vi "svfa_Mag to Mag2.vi"(0 "input signal":dbl[](array[numeric]) format="%.2f", 1 "power/magnitude desired":enum16{"no change", "power", "magnitude"}(ring), 5 "linear/dB":enum16{"linear", "dB"}(ring), 7 "power/magnitude":enum16{"power", "magnitude"}(ring), 9 "view":enum16{"rms", "peak", "peak-peak"}(ring), 11 "dB reference":dbl format="%.2f") -> (4 "converted signal":dbl[](array[numeric]) format="%.2f", 6 "dup linear/dB":enum16{"linear", "dB"}(ring), 8 "power/magnitude (out)":enum16{"power", "magnitude"}(ring), 10 "dup view":enum16{"rms", "peak", "peak-peak"}(ring), 15 "dB reference (out)":dbl format="%.2f")   [LabVIEW 2017]
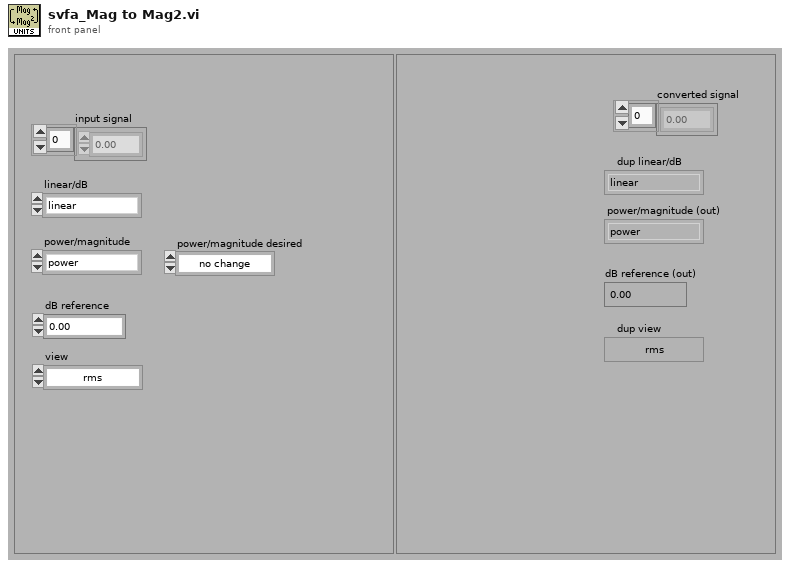
[diagram p1: front panel]
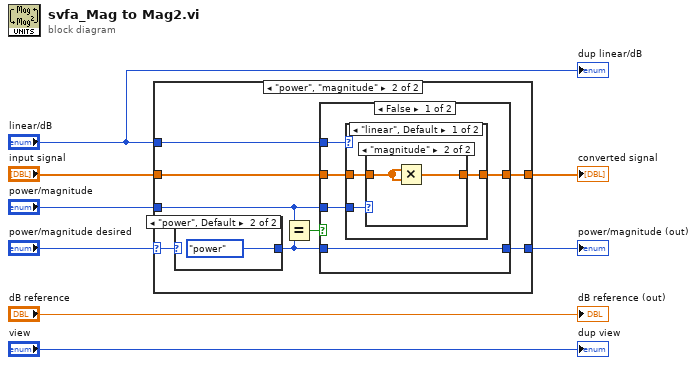
[diagram p0: block diagram]
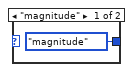
[diagram p3: hidden frame]
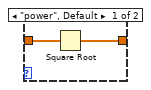
[diagram p4: hidden frame]
diagram:
  n1 = case shown="\"power\", \"magnitude\"" "power/magnitude desired" {
    selector: "power/magnitude desired" -> [_ w13]
    tunnel: [w9 w18] -> w8
    tunnel: [w10 w17] -> w7
    tunnel: "linear/dB" -> [_ w16]
    tunnel: "power/magnitude" -> [w9 w11]
    tunnel: "input signal" -> [w10 w15]
    frame "no change", Default {
    }
    frame "power", "magnitude" {
      n2 = case shown="\"power\", Default" w13 {
        tunnel: [enum16{"power", "magnitude"}."magnitude" ("power/magnitude") enum16{"power", "magnitude"}."power" ("power/magnitude")] -> w12
        frame "magnitude" {
        }
        frame "power", Default {
        }
      }
      n3 = Equal?(x=w11, y=w12) -> (x = y?=w14:bool)
      n4 = case shown="False" w14 {
        tunnel: w15 -> [w24 w35]
        tunnel: [w23 w35] -> w17
        tunnel: w16 -> [w25 _]
        tunnel: [w22 w34] -> w18
        tunnel: w12 -> [w22 w34]
        tunnel: w11 -> [w21 _]
        frame False {
          n5 = case shown="\"linear\", Default" w25 {
            tunnel: w24 -> [w28 w33]
            tunnel: [w27 w33] -> w23
            tunnel: w21 -> [w26 _]
            frame "linear", Default {
              n6 = case shown="\"magnitude\"" w26 {
                tunnel: w28 -> [w29 w32]
                tunnel: [w30 w31] -> w27
                frame "power", Default {
                  n7 = Square Root(x=w29) -> (sqrt(x)=w30:dbl[])
                }
                frame "magnitude" {
                  n8 = Multiply(x=w32, y=w32) -> (x*y=w31:dbl[])
                }
              }
            }
            frame "dB" {
            }
          }
        }
        frame True {
        }
      }
    }
  }
  "power/magnitude (out)" <- w8
  "converted signal" <- w7
  "dup linear/dB" <- "linear/dB"
  "dup view" <- "view"
  "dB reference (out)" <- "dB reference"
